vi "STD设置用户校准参数.vi"(7 "探头":T1(ring), 8 "error in (no error)":errorcluster caption="错误输入（无错误）", 10 "用户校准参数":cluster{"K":sgl, "B":sgl}, 11 "MB session in":refnum<class "MB_Master.lvclass">) -> (0 "error out":errorcluster caption="错误输出", 3 "MB session out":refnum<class "MB_Master.lvclass">)   [LabVIEW 2016, in "斯坦道多参数.lvlib"]
uses:
  <vilib>/Plasmionique/MB Master/MB_Master/MB_Master.lvclass
  <vilib>/Plasmionique/MB Master/MB Master.lvlib
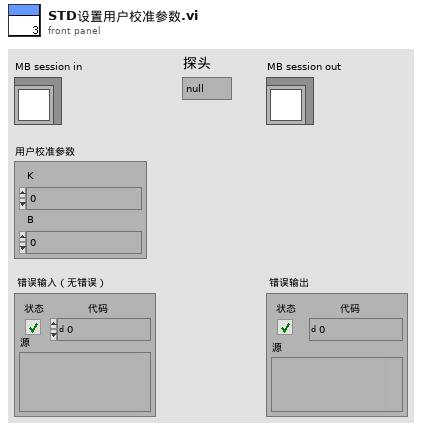
[diagram p1: front panel]
types:
  T1 = enum16{"null", "pH", "DO", "浊度", "电导率", "叶绿素a", "DO2", "藻密度"}
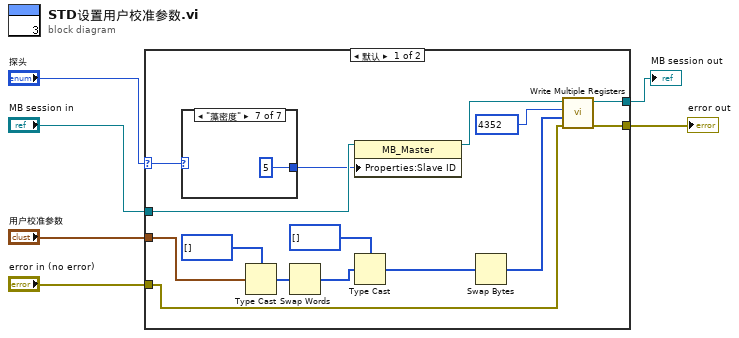
[diagram p0: block diagram]
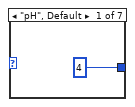
[diagram p2: hidden frame]
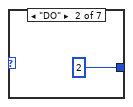
[diagram p3: hidden frame]
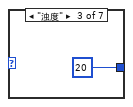
[diagram p4: hidden frame]
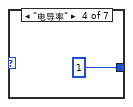
[diagram p5: hidden frame]
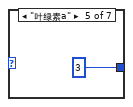
[diagram p6: hidden frame]
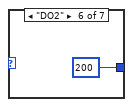
[diagram p7: hidden frame]
diagram:
  n1 = case shown="默认" "探头" {
    selector: "探头" -> [w7 _]
    tunnel: "error in (no error)" -> [w20 w29]
    tunnel: [w19 w29] -> w5
    tunnel: "用户校准参数" -> [w12 _]
    tunnel: "MB session in" -> [w10 w30]
    tunnel: [w8 w30] -> w2
    frame Default {
      n2 = case shown="\"藻密度\"" w7 {
        tunnel: [u16 4 ("y") u16 2 ("y") u16 20 ("y") u16 1 ("y") u16 3 ("y") u16 200 ("y") u16 5 ("y")] -> w9
        frame "pH", Default {
        }
        frame "DO" {
        }
        frame "浊度" {
        }
        frame "电导率" {
        }
        frame "叶绿素a" {
        }
        frame "DO2" {
        }
        frame "藻密度" {
        }
      }
      n3 = Type Cast(type=u32[] [] ("数组 2"), x=w12) -> (*(type *) &x=w11:u32[])
      n4 = Swap Words(1:w11) -> (0:w15:u32[])
      n5 = property class="MB_Master"(reference=w10, "Properties:Slave ID"=w9) -> (reference out=w18:refnum<class "MB_Master.lvclass">)  [unwired: 1 in, 1 out]
      n6 = Type Cast(type=u16[] [] ("数组 2"), x=w15) -> (*(type *) &x=w14:u16[])
      n7 = Swap Bytes(anything=w14) -> (byte swapped=w13:u16[])
      n8 = call <vilib>:"Write Multiple Registers.vi"("error in (no error)"=w20, "values"=w13, "starting address"=u16 4352, "MB session in"=w18) -> ("error out"=w19:errorcluster, "MB session out"=w8:refnum<class "MB_Master.lvclass">)  [unwired: 6 in]
    }
    frame "null" {
    }
  }
  "error out" <- w5
  "MB session out" <- w2
